vi "Send Log Data.vi"(8 "error in (no error)":errorcluster, 10 "Data":T1[](array[typedef]), 11 "Producer in":refnum<class "Log Producer.lvclass">) -> (0 "error out":errorcluster, 3 "Producer out":refnum<class "Log Producer.lvclass">)   [LabVIEW 2020, in "AIM ARINC 429 Engine.lvlib" / "Implementation.lvlib" / "Word Logging.lvlib"]
uses:
  Word Logging.lvlib
  Log Producer/Log Producer.lvclass
  Word.ctl
  Implementation.lvlib
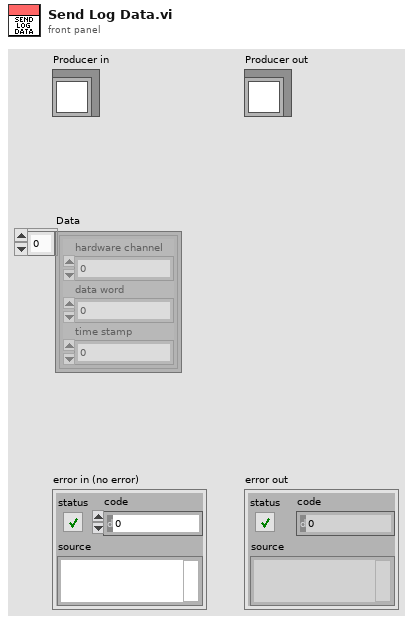
[diagram p1: front panel]
types:
  T1 = typedef "AIM ARINC 429 Engine.lvlib/Implementation.lvlib/Word.ctl" = cluster{"hardware channel":u8, "data word":u32, "time stamp":dbl}
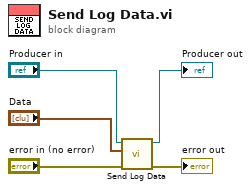
[diagram p0: block diagram]
diagram:
  n1 = call "Send Log Data.vi"("error in"="error in (no error)", "Data"="Data", "Log Producer in"="Producer in") -> ("error out"=→"error out":errorcluster, "Log Producer out"=→"Producer out":refnum<class "Log Producer.lvclass">)  [unwired: 7 in]
